vi "Set Downstream Job.vi"(8 "error in (no error)":errorcluster, 10 "Downstream Job":string, 11 "Build Job in":refnum<class "Build Job.lvclass">) -> (0 "error out":errorcluster, 3 "Build Job out":refnum<class "Build Job.lvclass">)   [LabVIEW 2014, in "Build Job.lvclass"]
uses:
  Build Job.lvclass
  Build Job.lvclass/Build Job.ctl
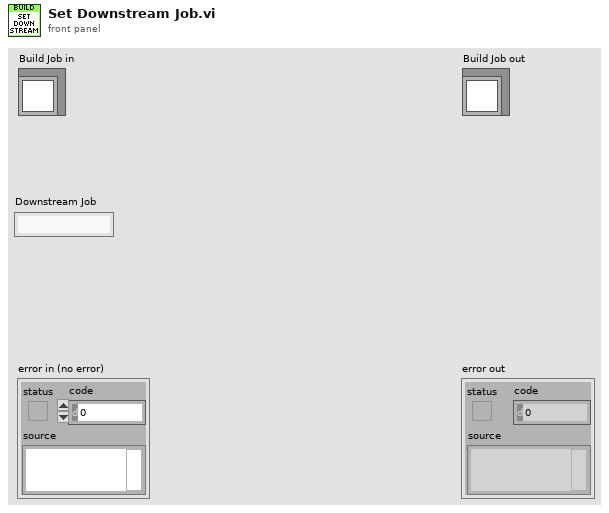
[diagram p1: front panel]
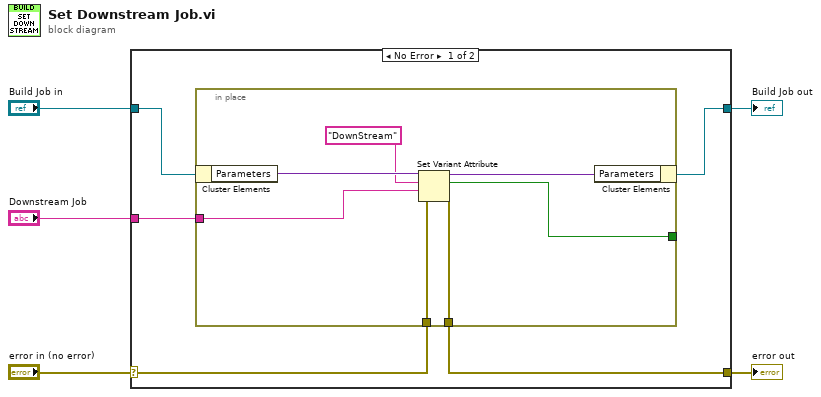
[diagram p0: block diagram]
diagram:
  n1 = case shown="No Error" "error in (no error)" {
    selector: "error in (no error)" -> [w8 w19]
    tunnel: [w7 w19] -> w4
    tunnel: [w9 w18] -> w2
    tunnel: "Build Job in" -> [w10 w18]
    tunnel: "Downstream Job" -> [w6 _]
    frame No Error {
      n2 = in-place {
        in-place-border: w8 -> [w14]
        in-place-border: [w13] -> w7
        in-place-border: w6 -> [w12]
        in-place-border: [w11] -> _
        n3 = in-place-cluster #1(w10) -> ("Parameters"=w17:variant)
        n4 = Set Variant Attribute(Variant=w17, name="DownStream", value=w12, error in=w14) -> (Variant out=w15:variant, replaced=w11:bool, error out=w13:errorcluster)
        n5 = in-place-cluster #1("Parameters"=w15) -> (w9:refnum<class "Build Job.lvclass">)
      }
    }
    frame Error {
    }
  }
  "error out" <- w4
  "Build Job out" <- w2
